vi "AndExpression.vi"(8 "error in (no error)":errorcluster, 9 "expr2":refnum<class "TerminalExpression.lvclass">, 10 "expr1":refnum<class "TerminalExpression.lvclass">, 11 "AndExpression in":refnum<class "AndExpression.lvclass">) -> (0 "error out":errorcluster, 3 "AndExpression out":refnum<class "AndExpression.lvclass">)   [LabVIEW 2018, in "AndExpression.lvclass"]
uses:
  AndExpression.lvclass
  TerminalExpression Class/TerminalExpression.lvclass
  AndExpression.lvclass/AndExpression.ctl
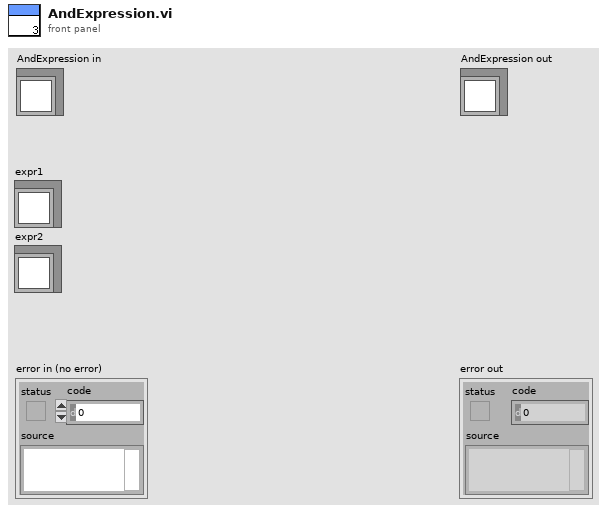
[diagram p1: front panel]
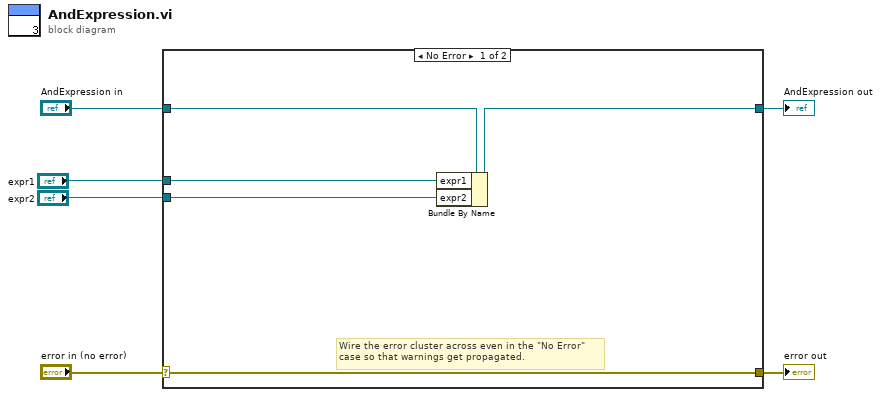
[diagram p0: block diagram]
diagram:
  n1 = case shown="No Error" "error in (no error)" {
    selector: "error in (no error)" -> [w10 w13]
    tunnel: [w10 w13] -> w5
    tunnel: [w9 w12] -> w3
    tunnel: "AndExpression in" -> [w11 w12]
    tunnel: "expr1" -> [w8 _]
    tunnel: "expr2" -> [w7 _]
    frame No Error {
      # "Wire the error cluster across even in the \"No Error\"\ncase so that warnings get propagated."
      n2 = Bundle By Name(cluster=w11, "expr1"=w8, "expr2"=w7) -> (w9:refnum<class "AndExpression.lvclass">)
    }
    frame Error {
    }
  }
  "error out" <- w5
  "AndExpression out" <- w3
